vi "wait on daemon.vi"(11 "daemons":refnum<vi>[](array[refnum])) -> (0 "error out":errorcluster)   [LabVIEW 2013, in "TBM module execution interface.lvclass"]
uses:
  TBM module execution interface.lvclass
  <vilib>/NI/Tag Bus/data stream/publisher/publisher.lvclass
  <vilib>/NI/Tag Bus/data stream/subscriber/subscriber.lvclass
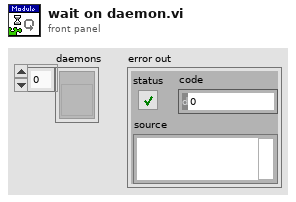
[diagram p1: front panel]
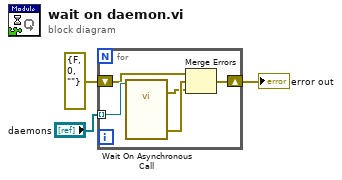
[diagram p0: block diagram]
diagram:
  n1 = for {
    tunnel: "daemons" -> [w8] mode=indexing
    shift-right: [w5] -> w1
    shift-left: errorcluster {"status"=FALSE, "code"=0, "source"=""} ("error IO") -> [w4]
    n2 = call-by-ref "Wait On Asynchronous Call"(reference=w8) -> (error out=w6:errorcluster, 0:"error out"=w7:errorcluster)  [unwired: 12 in, 1 out]
    n3 = Merge Errors(w4, w7, w6) -> (w5:errorcluster)
  }
  "error out" <- w1
